vi "Delete_First_Rows.vi"(0 "File Type":string, 1 "Data In":string[][](array[string])) -> (2 "Rows removed":i32, 3 "Deleted Rows":string[][](array[string]), 4 "Data Out":string[][](array[string]))   [LabVIEW 2021]
panel:
  # "#WatchOut! If more than 50% of an upper row is blank, it will be trimmed off, thinking it's 4th row title"
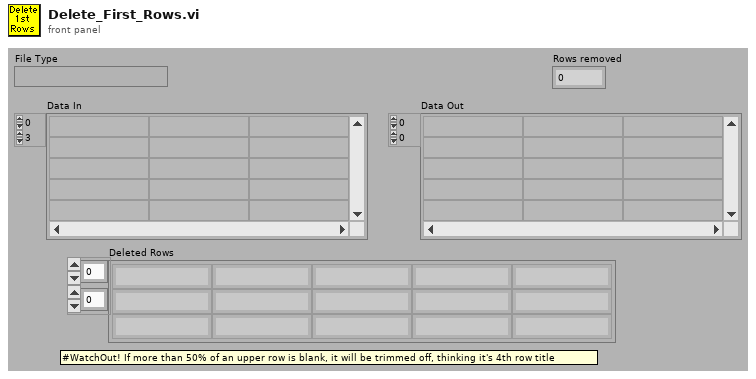
[diagram p1: front panel]
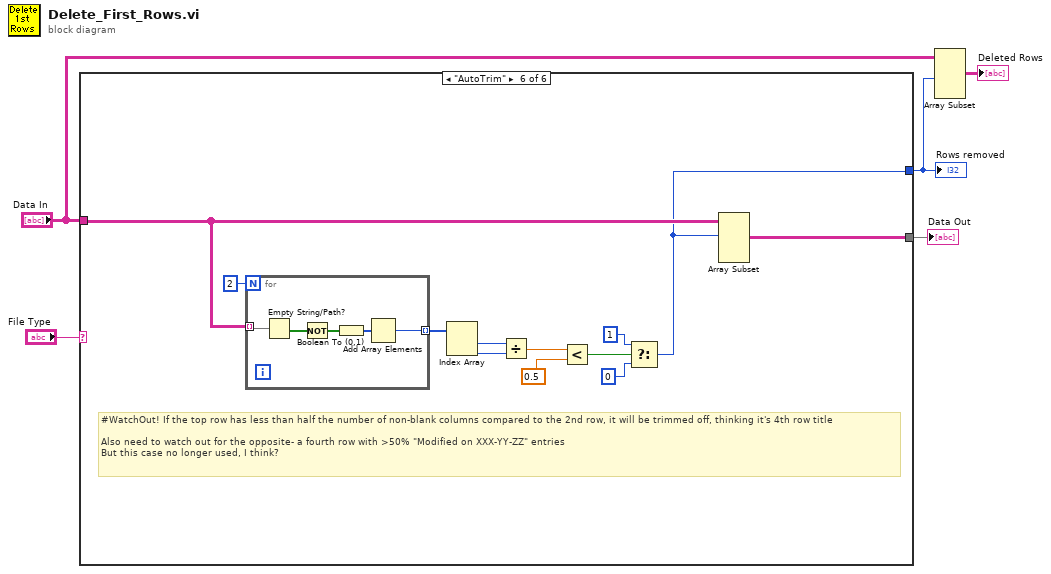
[diagram p0: block diagram]
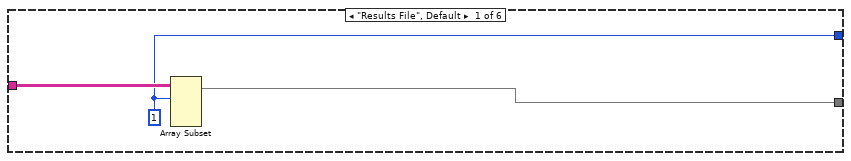
[diagram p2: hidden frame]
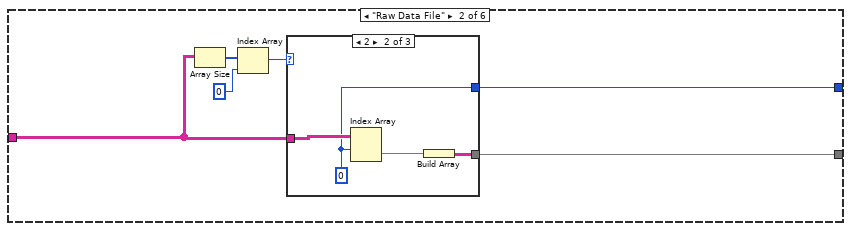
[diagram p3: hidden frame]
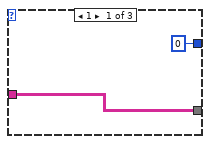
[diagram p4: hidden frame]
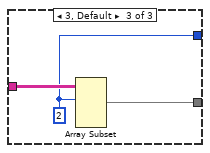
[diagram p5: hidden frame]
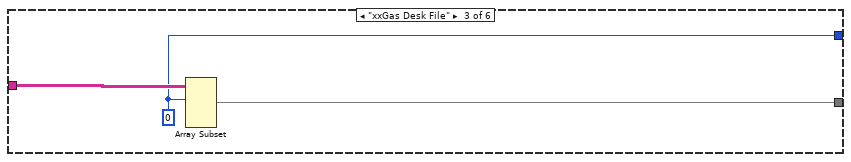
[diagram p6: hidden frame]
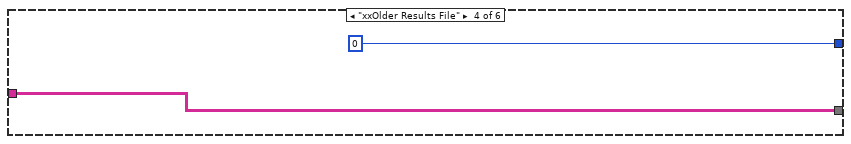
[diagram p7: hidden frame]
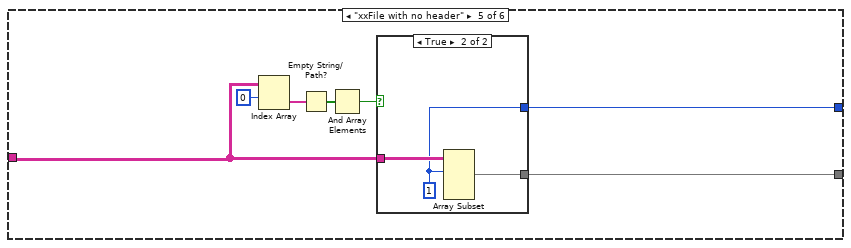
[diagram p8: hidden frame]
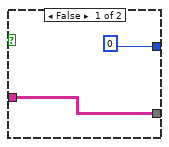
[diagram p9: hidden frame]
diagram:
  n1 = case shown="\"AutoTrim\"" "File Type" {
    tunnel: [w7 w14 w25 w28 w31 w52] -> w5
    tunnel: "Data In" -> [w8 w12 w26 w28 w32 w50]
    tunnel: [w6 w9 w24 0 ("Array Index") w29 w43] -> w2
    frame "Results File", Default {
      w6 = 1 ("Array Index")
      n2 = Array Subset(array=w8, index (row)=w6) -> (w7:string[][])  [unwired: 3 in]
    }
    frame "Raw Data File" {
      n3 = Array Size(array=w12) -> (size(s)=w13:i32[])
      n4 = Index Array(array=w13, index=0 ("Index")) -> (element=w10:i32)
      n5 = case shown="2" w10 {
        tunnel: [w16 w18 w23] -> w14
        tunnel: w12 -> [w16 w20 w22]
        tunnel: [0 w17 w21] -> w9
        frame 1 {
        }
        frame 2 {
          w17 = 0 ("Index")
          n6 = Index Array(array=w20, index (row)=w17) -> (element=w19:string[])  [unwired: 1 in]
          n7 = Build Array(w19) -> (w18:string[][])
        }
        frame 3, Default {
          w21 = 2 ("Array Index")
          n8 = Array Subset(array=w22, index (row)=w21) -> (w23:string[][])  [unwired: 3 in]
        }
      }
    }
    frame "xxGas Desk File" {
      w24 = 0 ("Array Index")
      n9 = Array Subset(array=w26, index (row)=w24) -> (w25:string[][])  [unwired: 3 in]
    }
    frame "xxOlder Results File" {
    }
    frame "xxFile with no header" {
      n10 = Index Array(array=w32, index (row)=0) -> (element=w34:string[])  [unwired: 1 in]
      n11 = Empty String/Path?(string/path=w34) -> (empty?=w33:bool[])
      n12 = And Array Elements(Boolean array=w33) -> (logical AND=w30:bool)
      n13 = case shown="True" w30 {
        tunnel: w32 -> [w36 w40]
        tunnel: [w36 w39] -> w31
        tunnel: [0 ("Array Index") w38] -> w29
        frame False {
        }
        frame True {
          w38 = 1 ("Array Index")
          n14 = Array Subset(array=w40, index (row)=w38) -> (w39:string[][])  [unwired: 3 in]
        }
      }
    }
    frame "AutoTrim" {
      # "#WatchOut! If the top row has less than half the number of non-blank columns compared to the 2nd row, it will be trimmed off, thinking it's 4th row title\n\nAlso need to watch out for the opposite- a fourth row with >50% \"Modified on XXX-YY-ZZ\" entries\nBut this case no longer used, I think?"
      n15 = for {
        N: 2 -> [_]
        tunnel: w50 -> [w54] mode=indexing
        tunnel: [w55] -> w49 mode=indexing
        n16 = Empty String/Path?(string/path=w54) -> (empty?=w56:bool[])
        n17 = Not(x=w56) -> (.not. x?=w53:bool[])
        n18 = Boolean To (0,1)(Boolean=w53) -> (0, 1=w57:i16[])
        n19 = Add Array Elements(numeric array=w57) -> (sum=w55:i16)
      }
      n20 = Index Array(array=w49) -> (element #1=w48:i16, element #2=w47:i16)  [unwired: 2 in]
      n21 = Divide(x=w48, y=w47) -> (x/y=w46:dbl)
      n22 = Less?(x=w46, y=0.5) -> (x < y?=w44:bool)
      n23 = Select(t=1 ("Rows removed"), s=w44, f=0 ("Rows removed")) -> (s? t:f=w43:i32)
      n24 = Array Subset(array=w50, index (row)=w43) -> (w52:string[][])  [unwired: 3 in]
    }
  }
  "Data Out" <- w5
  "Rows removed" <- w2
  n25 = Array Subset(array="Data In", length (row)=w2) -> (→"Deleted Rows":string[][])  [unwired: 3 in]
